vi "recordStartPauseTime.vi"(8 "error in (no error)":errorcluster, 11 "Model in":refnum<class "Model.lvclass">) -> (0 "error out":errorcluster, 3 "Model out":refnum<class "Model.lvclass">)   [LabVIEW 2015]
uses:
  ApplicationElements/TestMonitor/TestMonitor.lvclass
  Model.lvclass
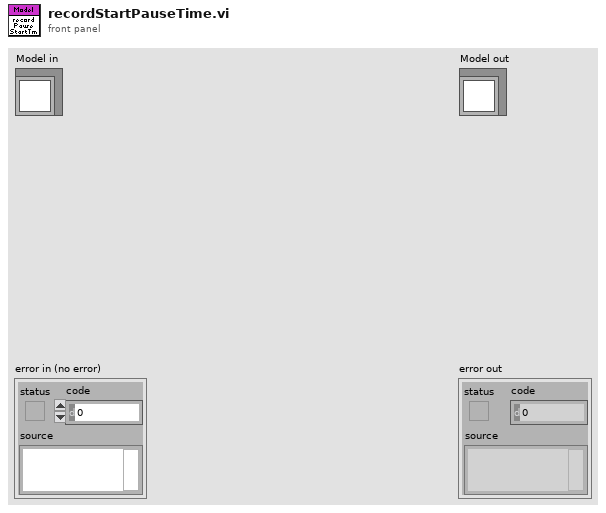
[diagram p1: front panel]
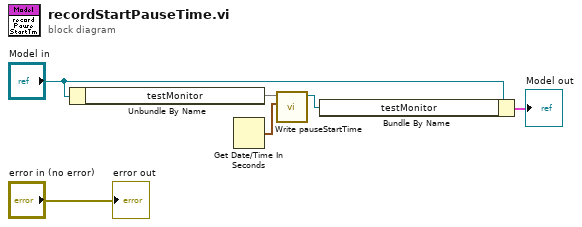
[diagram p0: block diagram]
diagram:
  n1 = Unbundle By Name("Model in") -> ("testMonitor"=w3)
  n2 = Get Date/Time In Seconds() -> (seconds since 1Jan1904=w1:timestamp)
  n3 = call "Write pauseStartTime.vi"("pauseStartTime"=w1, "TestMonitor in"=w3) -> ("TestMonitor out"=w2:refnum<class "TestMonitor.lvclass">)  [unwired: 9 in]
  n4 = Bundle By Name(cluster="Model in", "testMonitor"=w2) -> (→"Model out":cluster{})
  "error out" <- "error in (no error)"
